vi "Digilens DLP Gen2 UI .vi"(11 "TopLevel In":refnum<class "TopLevel.lvclass">) -> (3 "TopLevel Out":refnum<class "TopLevel.lvclass">)   [LabVIEW 2022 SP3, in "TopLevel.lvclass"] (continued)
              frame "Stage Head3", "Stage Head3 2" {
                n548 = Unbundle By Name(w1508) -> ("Prime Names.Prime 3"=w1507:string)
              }
              frame "Stage Head4", "Stage Head4 2" {
                n549 = Unbundle By Name(w1513) -> ("Prime Names.Prime 4"=w1512:string)
              }
              frame "Stage Head5", "Stage Head5 2" {
                n550 = Unbundle By Name(w1518) -> ("Prime Names.Prime 5"=w1517:string)
              }
              frame "Stage Head6", "Stage Head6 2" {
                n551 = Unbundle By Name(w1523) -> ("Prime Names.Prime 6"=w1522:string)
              }
            }
            n552 = Unbundle By Name(w1488) -> ("Motor Controller"=w1475:refnum<class "Motor Controller.lvclass">, "Methods:Accessors:ConfigDict"=w1487:T16)
            n553 = call <vilib>:"Get Dynamic CVT Data.vi"("error in (no error)"=w1486, "default value (empty variant)"=w1483, "DataName"=w1485, "dCVT DVR"=w1487) -> ("error out"=w1482:errorcluster, "value"=w1484:variant)  [unwired: 4 in, 2 out]
            n554 = Variant To Data(error in=w1482, type=w1483, Variant=w1484) -> (data=w1481:T27, error out=w1474:errorcluster)
            n555 = Unbundle By Name(w1481) -> ("PrimingMode"=w1480:T13)
            n556 = Equal?(x=w1480, y=PurgeMode--Enum."Purge") -> (x = y?=w1466:bool)
            n557 = Select(t=w1468, s=w1466, f=w1467) -> (s? t:f=w1469:i32)
            n558 = Bundle By Name(cluster=T20 {"Motor Controller Parameter"=enum."Move Stage to Under PH1", "value"=11} ("SetExplicitMessage API Data"), "value"=w1469, "Motor Controller Parameter"=w1471) -> (w1470:T20)
            n559 = Bundle By Name(cluster=T23 {"Command"=enum."GetExplicitMessage", "Arguments"="", "Data"=variant} ("API Command Cluster"), "Command"=API_Command_Enum."SetExplicitMessage", "Data"=w1470) -> (w1478:T23)
            n560 = call-dynamic "GenerateAPIEvent_Motor Controller.vi"("error in (no error)"=w1474, "API Command Cluster"=w1478, "Motor Controller In"=w1475) -> ("error out"=w1473:errorcluster)  [unwired: 6 in, 2 out]
          }
          event "Prime Interval 1", "Prime Duration 1", "Prime Repeats 1", "Freq 1": Value Change {
            n561 = event-data() -> ()  [unwired: 1 in, 6 out]
            n562 = Unbundle By Name(w1534) -> ("TopLevel out"=w1524:refnum<class "TopLevel.lvclass">, "Methods:Accessors:ConfigDict"=w1532:T16, "Prime Names.Prime 1"=w1531:string)
            n563 = call <vilib>:"Get Dynamic CVT Data.vi"("error in (no error)"=w1530, "default value (empty variant)"=T27 {"Interval (s)"=0.1, "PurgeDuration (s)"=0.1, "Repeats"=0, "PrimingMode"=enum."Pre-Purge", "Head"=enum."1", "Frequency (Hz)"=0, "PrintWeight"=0.1} ("Pre Purge API Data"), "DataName"=w1531, "dCVT DVR"=w1532) -> ("error out"=w1529:errorcluster, "found"=w1526:bool, "value"=w1528:variant, "dCVT DVR out"=w1525:T16)  [unwired: 4 in]
            n564 = case shown="True" w1526 {
              tunnel: w1531 -> [_ w1550]
              tunnel: [w1538 w1546] -> w1535
              tunnel: w1534 -> [w1539 w1545]
              tunnel: [w1539 w1544] -> w1533
              tunnel: w1529 -> [w1538 w1555]
              tunnel: w1528 -> [_ w1554]
              tunnel: w1525 -> [_ w1552]
              tunnel: w1524 -> [_ w1543]
              frame False {
              }
              frame True {
                n565 = Variant To Data(error in=w1555, type=T27 {"Interval (s)"=0.1, "PurgeDuration (s)"=0.1, "Repeats"=0, "PrimingMode"=enum."Pre-Purge", "Head"=enum."1", "Frequency (Hz)"=0, "PrintWeight"=0.1} ("Pre Purge API Data"), Variant=w1554) -> (data=w1553:T27, error out=w1547:errorcluster)
                n566 = Bundle By Name(cluster=w1553, "Interval (s)"="Prime Interval 1", "PurgeDuration (s)"="Prime Duration 1", "Repeats"="Prime Repeats 1", "PrimingMode"="Prime Mode 1", "Frequency (Hz)"="Freq 1") -> (w1549:T27)
                n567 = call <vilib>:"Set Dynamic CVT Data.vi"("error in (no error)"=w1547, "value"=w1549, "DataName"=w1550, "dCVT DVR"=w1552) -> ("error out"=w1548:errorcluster, "dCVT DVR out"=w1551:T16)  [unwired: 5 in, 1 out]
                n568 = call-dynamic "Write ConfigDict.vi"("error in (no error)"=w1548, "ConfigDIct"=w1551, "TopLevel in"=w1543) -> ("error out"=w1546:errorcluster, "TopLevel out"=w1542:refnum<class "TopLevel.lvclass">)  [unwired: 7 in]
                n569 = Bundle By Name(cluster=w1545, "TopLevel out"=w1542) -> (w1544:T77)
              }
            }
          }
          event "Prime Interval 2", "Prime Duration 2", "Prime Repeats 2", "Freq 2": Value Change {
            n570 = event-data() -> ()  [unwired: 1 in, 6 out]
            n571 = Unbundle By Name(w1568) -> ("TopLevel out"=w1560:refnum<class "TopLevel.lvclass">, "Methods:Accessors:ConfigDict"=w1567:T16, "Prime Names.Prime 2"=w1566:string)
            n572 = call <vilib>:"Get Dynamic CVT Data.vi"("error in (no error)"=w1571, "default value (empty variant)"=T27 {"Interval (s)"=0.1, "PurgeDuration (s)"=0.1, "Repeats"=0, "PrimingMode"=enum."Pre-Purge", "Head"=enum."1", "Frequency (Hz)"=0, "PrintWeight"=0.1} ("Pre Purge API Data"), "DataName"=w1566, "dCVT DVR"=w1567) -> ("error out"=w1565:errorcluster, "found"=w1562:bool, "value"=w1564:variant, "dCVT DVR out"=w1561:T16)  [unwired: 4 in]
            n573 = case shown="True" w1562 {
              tunnel: w1566 -> [_ w1590]
              tunnel: [w1574 w1586] -> w1570
              tunnel: w1568 -> [w1575 w1585]
              tunnel: [w1575 w1584] -> w1569
              tunnel: w1565 -> [w1574 w1595]
              tunnel: w1564 -> [_ w1594]
              tunnel: w1561 -> [_ w1592]
              tunnel: w1560 -> [_ w1583]
              frame False {
              }
              frame True {
                n574 = Variant To Data(error in=w1595, type=T27 {"Interval (s)"=0.1, "PurgeDuration (s)"=0.1, "Repeats"=0, "PrimingMode"=enum."Pre-Purge", "Head"=enum."1", "Frequency (Hz)"=0, "PrintWeight"=0.1} ("Pre Purge API Data"), Variant=w1594) -> (data=w1593:T27, error out=w1587:errorcluster)
                n575 = Bundle By Name(cluster=w1593, "Interval (s)"="Prime Interval 2", "PurgeDuration (s)"="Prime Duration 2", "Repeats"="Prime Repeats 2", "PrimingMode"="Prime Mode 2", "Frequency (Hz)"="Freq 2") -> (w1589:T27)
                n576 = call <vilib>:"Set Dynamic CVT Data.vi"("error in (no error)"=w1587, "value"=w1589, "DataName"=w1590, "dCVT DVR"=w1592) -> ("error out"=w1588:errorcluster, "dCVT DVR out"=w1591:T16)  [unwired: 5 in, 1 out]
                n577 = call-dynamic "Write ConfigDict.vi"("error in (no error)"=w1588, "ConfigDIct"=w1591, "TopLevel in"=w1583) -> ("error out"=w1586:errorcluster, "TopLevel out"=w1582:refnum<class "TopLevel.lvclass">)  [unwired: 7 in]
                n578 = Bundle By Name(cluster=w1585, "TopLevel out"=w1582) -> (w1584:T77)
              }
            }
          }
          event "Prime Interval 3", "Prime Duration 3", "Prime Repeats 3", "Freq 3": Value Change {
            n579 = event-data() -> ()  [unwired: 1 in, 6 out]
            n580 = Unbundle By Name(w1604) -> ("TopLevel out"=w1596:refnum<class "TopLevel.lvclass">, "Methods:Accessors:ConfigDict"=w1603:T16, "Prime Names.Prime 3"=w1602:string)
            n581 = call <vilib>:"Get Dynamic CVT Data.vi"("error in (no error)"=w1607, "default value (empty variant)"=T27 {"Interval (s)"=0.1, "PurgeDuration (s)"=0.1, "Repeats"=0, "PrimingMode"=enum."Pre-Purge", "Head"=enum."1", "Frequency (Hz)"=0, "PrintWeight"=0.1} ("Pre Purge API Data"), "DataName"=w1602, "dCVT DVR"=w1603) -> ("error out"=w1601:errorcluster, "found"=w1598:bool, "value"=w1600:variant, "dCVT DVR out"=w1597:T16)  [unwired: 4 in]
            n582 = case shown="True" w1598 {
              tunnel: w1602 -> [_ w1626]
              tunnel: [w1610 w1622] -> w1606
              tunnel: w1604 -> [w1611 w1621]
              tunnel: [w1611 w1620] -> w1605
              tunnel: w1601 -> [w1610 w1631]
              tunnel: w1600 -> [_ w1630]
              tunnel: w1597 -> [_ w1628]
              tunnel: w1596 -> [_ w1619]
              frame False {
              }
              frame True {
                n583 = Variant To Data(error in=w1631, type=T27 {"Interval (s)"=0.1, "PurgeDuration (s)"=0.1, "Repeats"=0, "PrimingMode"=enum."Pre-Purge", "Head"=enum."1", "Frequency (Hz)"=0, "PrintWeight"=0.1} ("Pre Purge API Data"), Variant=w1630) -> (data=w1629:T27, error out=w1623:errorcluster)
                n584 = Bundle By Name(cluster=w1629, "Interval (s)"="Prime Interval 3", "PurgeDuration (s)"="Prime Duration 3", "Repeats"="Prime Repeats 3", "PrimingMode"="Prime Mode 3", "Frequency (Hz)"="Freq 3") -> (w1625:T27)
                n585 = call <vilib>:"Set Dynamic CVT Data.vi"("error in (no error)"=w1623, "value"=w1625, "DataName"=w1626, "dCVT DVR"=w1628) -> ("error out"=w1624:errorcluster, "dCVT DVR out"=w1627:T16)  [unwired: 5 in, 1 out]
                n586 = call-dynamic "Write ConfigDict.vi"("error in (no error)"=w1624, "ConfigDIct"=w1627, "TopLevel in"=w1619) -> ("error out"=w1622:errorcluster, "TopLevel out"=w1618:refnum<class "TopLevel.lvclass">)  [unwired: 7 in]
                n587 = Bundle By Name(cluster=w1621, "TopLevel out"=w1618) -> (w1620:T77)
              }
            }
          }
          event "Prime Interval 4", "Prime Duration 4", "Prime Repeats 4", "Freq 4": Value Change {
            n588 = event-data() -> ()  [unwired: 1 in, 6 out]
            n589 = Unbundle By Name(w1640) -> ("TopLevel out"=w1632:refnum<class "TopLevel.lvclass">, "Methods:Accessors:ConfigDict"=w1639:T16, "Prime Names.Prime 4"=w1638:string)
            n590 = call <vilib>:"Get Dynamic CVT Data.vi"("error in (no error)"=w1643, "default value (empty variant)"=T27 {"Interval (s)"=0.1, "PurgeDuration (s)"=0.1, "Repeats"=0, "PrimingMode"=enum."Pre-Purge", "Head"=enum."1", "Frequency (Hz)"=0, "PrintWeight"=0.1} ("Pre Purge API Data"), "DataName"=w1638, "dCVT DVR"=w1639) -> ("error out"=w1637:errorcluster, "found"=w1634:bool, "value"=w1636:variant, "dCVT DVR out"=w1633:T16)  [unwired: 4 in]
            n591 = case shown="True" w1634 {
              tunnel: w1638 -> [_ w1662]
              tunnel: [w1646 w1658] -> w1642
              tunnel: w1640 -> [w1647 w1657]
              tunnel: [w1647 w1656] -> w1641
              tunnel: w1637 -> [w1646 w1667]
              tunnel: w1636 -> [_ w1666]
              tunnel: w1633 -> [_ w1664]
              tunnel: w1632 -> [_ w1655]
              frame False {
              }
              frame True {
                n592 = Variant To Data(error in=w1667, type=T27 {"Interval (s)"=0.1, "PurgeDuration (s)"=0.1, "Repeats"=0, "PrimingMode"=enum."Pre-Purge", "Head"=enum."1", "Frequency (Hz)"=0, "PrintWeight"=0.1} ("Pre Purge API Data"), Variant=w1666) -> (data=w1665:T27, error out=w1659:errorcluster)
                n593 = Bundle By Name(cluster=w1665, "Interval (s)"="Prime Interval 4", "PurgeDuration (s)"="Prime Duration 4", "Repeats"="Prime Repeats 4", "PrimingMode"="Prime Mode 4", "Frequency (Hz)"="Freq 4") -> (w1661:T27)
                n594 = call <vilib>:"Set Dynamic CVT Data.vi"("error in (no error)"=w1659, "value"=w1661, "DataName"=w1662, "dCVT DVR"=w1664) -> ("error out"=w1660:errorcluster, "dCVT DVR out"=w1663:T16)  [unwired: 5 in, 1 out]
                n595 = call-dynamic "Write ConfigDict.vi"("error in (no error)"=w1660, "ConfigDIct"=w1663, "TopLevel in"=w1655) -> ("error out"=w1658:errorcluster, "TopLevel out"=w1654:refnum<class "TopLevel.lvclass">)  [unwired: 7 in]
                n596 = Bundle By Name(cluster=w1657, "TopLevel out"=w1654) -> (w1656:T77)
              }
            }
          }
          event "Prime Interavl 5", "Prime Duration 5", "Prime Repeats 5", "Freq 5": Value Change {
            n597 = event-data() -> ()  [unwired: 1 in, 6 out]
            n598 = Unbundle By Name(w1676) -> ("TopLevel out"=w1668:refnum<class "TopLevel.lvclass">, "Methods:Accessors:ConfigDict"=w1675:T16, "Prime Names.Prime 5"=w1674:string)
            n599 = call <vilib>:"Get Dynamic CVT Data.vi"("error in (no error)"=w1679, "default value (empty variant)"=T27 {"Interval (s)"=0.1, "PurgeDuration (s)"=0.1, "Repeats"=0, "PrimingMode"=enum."Pre-Purge", "Head"=enum."1", "Frequency (Hz)"=0, "PrintWeight"=0.1} ("Pre Purge API Data"), "DataName"=w1674, "dCVT DVR"=w1675) -> ("error out"=w1673:errorcluster, "found"=w1670:bool, "value"=w1672:variant, "dCVT DVR out"=w1669:T16)  [unwired: 4 in]
            n600 = case shown="True" w1670 {
              tunnel: w1674 -> [_ w1698]
              tunnel: [w1682 w1694] -> w1678
              tunnel: w1676 -> [w1683 w1693]
              tunnel: [w1683 w1692] -> w1677
              tunnel: w1673 -> [w1682 w1703]
              tunnel: w1672 -> [_ w1702]
              tunnel: w1669 -> [_ w1700]
              tunnel: w1668 -> [_ w1691]
              frame False {
              }
              frame True {
                n601 = Variant To Data(error in=w1703, type=T27 {"Interval (s)"=0.1, "PurgeDuration (s)"=0.1, "Repeats"=0, "PrimingMode"=enum."Pre-Purge", "Head"=enum."1", "Frequency (Hz)"=0, "PrintWeight"=0.1} ("Pre Purge API Data"), Variant=w1702) -> (data=w1701:T27, error out=w1695:errorcluster)
                n602 = Bundle By Name(cluster=w1701, "Interval (s)"="Prime Interavl 5", "PurgeDuration (s)"="Prime Duration 5", "Repeats"="Prime Repeats 5", "PrimingMode"="Prime Mode 5", "Frequency (Hz)"="Freq 5") -> (w1697:T27)
                n603 = call <vilib>:"Set Dynamic CVT Data.vi"("error in (no error)"=w1695, "value"=w1697, "DataName"=w1698, "dCVT DVR"=w1700) -> ("error out"=w1696:errorcluster, "dCVT DVR out"=w1699:T16)  [unwired: 5 in, 1 out]
                n604 = call-dynamic "Write ConfigDict.vi"("error in (no error)"=w1696, "ConfigDIct"=w1699, "TopLevel in"=w1691) -> ("error out"=w1694:errorcluster, "TopLevel out"=w1690:refnum<class "TopLevel.lvclass">)  [unwired: 7 in]
                n605 = Bundle By Name(cluster=w1693, "TopLevel out"=w1690) -> (w1692:T77)
              }
            }
          }
          event "Prime Interval 6", "Prime Duration 6", "Prime Repeats 6": Value Change {
            n606 = event-data() -> ()  [unwired: 1 in, 6 out]
            n607 = Unbundle By Name(w1712) -> ("TopLevel out"=w1704:refnum<class "TopLevel.lvclass">, "Methods:Accessors:ConfigDict"=w1711:T16, "Prime Names.Prime 6"=w1710:string)
            n608 = call <vilib>:"Get Dynamic CVT Data.vi"("error in (no error)"=w1715, "default value (empty variant)"=T27 {"Interval (s)"=0.1, "PurgeDuration (s)"=0.1, "Repeats"=0, "PrimingMode"=enum."Pre-Purge", "Head"=enum."1", "Frequency (Hz)"=0, "PrintWeight"=0.1} ("Pre Purge API Data"), "DataName"=w1710, "dCVT DVR"=w1711) -> ("error out"=w1709:errorcluster, "found"=w1706:bool, "value"=w1708:variant, "dCVT DVR out"=w1705:T16)  [unwired: 4 in]
            n609 = case shown="True" w1706 {
              tunnel: w1710 -> [_ w1734]
              tunnel: [w1719 w1730] -> w1714
              tunnel: w1709 -> [w1719 w1739]
              tunnel: w1708 -> [_ w1738]
              tunnel: w1705 -> [_ w1736]
              tunnel: w1704 -> [_ w1729]
              tunnel: w1712 -> [w1718 w1722]
              tunnel: [w1718 w1721] -> w1713
              frame False {
              }
              frame True {
                n610 = Variant To Data(error in=w1739, type=T27 {"Interval (s)"=0.1, "PurgeDuration (s)"=0.1, "Repeats"=0, "PrimingMode"=enum."Pre-Purge", "Head"=enum."1", "Frequency (Hz)"=0, "PrintWeight"=0.1} ("Pre Purge API Data"), Variant=w1738) -> (data=w1737:T27, error out=w1731:errorcluster)
                n611 = Bundle By Name(cluster=w1737, "Interval (s)"="Prime Interval 6", "PurgeDuration (s)"="Prime Duration 6", "Repeats"="Prime Repeats 6", "PrimingMode"="Prime Mode 6", "Frequency (Hz)"="Freq 6") -> (w1733:T27)
                n612 = call <vilib>:"Set Dynamic CVT Data.vi"("error in (no error)"=w1731, "value"=w1733, "DataName"=w1734, "dCVT DVR"=w1736) -> ("error out"=w1732:errorcluster, "dCVT DVR out"=w1735:T16)  [unwired: 5 in, 1 out]
                n613 = call-dynamic "Write ConfigDict.vi"("error in (no error)"=w1732, "ConfigDIct"=w1735, "TopLevel in"=w1729) -> ("error out"=w1730:errorcluster, "TopLevel out"=w1728:refnum<class "TopLevel.lvclass">)  [unwired: 7 in]
                n614 = Bundle By Name(cluster=w1722, "TopLevel out"=w1728) -> (w1721:T77)
              }
            }
          }
          event "Print": Value Change {
            n615 = event-data() -> ()  [unwired: 1 in, 6 out]
            n616 = Bundle By Name(cluster=T28 {"Command File Path"=path "", "No. of Print Repeats"=1, "HomeOnComplete"=FALSE}, "Command File Path"="Command File Path", "No. of Print Repeats"="Print Passes", "HomeOnComplete"="HomeOnComplete") -> (w1744:T28)
            n617 = Bundle By Name(cluster=T29 {"Command"=enum."Execute Printer Commands", "Arguments"="", "Data"=variant} ("API Command Cluster"), "Command"=API_Command_Enum."Execute Printer Commands", "Data"=w1744) -> (w1748:T29)
            n618 = call-dynamic "GenerateAPIEvent_TopLevel.vi"("Wait (F)"=FALSE, "error in (no error)"=w1750, "API Command Cluster"=w1748, "TopLevel in"=w1752) -> ("error out"=w1751:errorcluster, "TopLevel out"=w1753:refnum<class "TopLevel.lvclass">)  [unwired: 6 in]
          }
          event "IdlePrint": Value Change {
            n619 = event-data() -> ("NewVal"=w1758:bool)  [unwired: 1 in, 5 out]
            n620 = case shown="True" w1758 {
              tunnel: [API_Command_Enum."StopIdlePrintCycle" ("Command") API_Command_Enum."ExecuteIdlePrintCycle" ("Command")] -> w1762
              tunnel: [w1771 w1779] -> w1761
              tunnel: w1758 -> [_ w1776]
              tunnel: ["UI: SetUIControlsState>>enable" ("State(s) in Front (\"\")") "UI: SetUIControlsState>>disable" ("State(s) in Front (\"\")")] -> w1755
              frame False {
                n621 = Bundle By Name(cluster=T30 {"Command File Path"=path "", "IdleMode"=FALSE, "IdleCycleInterval(s)"=0.0} ("Cluster"), "IdleMode"=FALSE) -> (w1771:T30)
              }
              frame True {
                n622 = property on="Command File Path" class="Path"() -> ("Value"=w1775:path)  [unwired: 2 in, 2 out]
                n623 = Bundle By Name(cluster=T30 {"Command File Path"=path "", "IdleMode"=FALSE, "IdleCycleInterval(s)"=0.0} ("Cluster"), "Command File Path"=w1775, "IdleMode"=w1776, "IdleCycleInterval(s)"="Idle Intervals (s)") -> (w1779:T30)
              }
            }
            n624 = Bundle By Name(cluster=T29 {"Command"=enum."Execute Printer Commands", "Arguments"="", "Data"=variant} ("API Command Cluster"), "Command"=w1762, "Data"=w1761) -> (w1763:T29)
            n625 = call-dynamic "GenerateAPIEvent_TopLevel.vi"("Wait (F)"=FALSE, "error in (no error)"=w1765, "API Command Cluster"=w1763, "TopLevel in"=w1767) -> ("error out"=w1766:errorcluster, "TopLevel out"=w1768:refnum<class "TopLevel.lvclass">)  [unwired: 6 in]
            n626 = call <vilib>:"Add State(s) to Queue__JKI_lib_State_Machine.vi"("State(s) in Front (\"\")"=w1755, "State(s) in (\"\")"=w1756) -> ("States Out"=w1757:string)  [unwired: 13 in]
          }
          event User Event {
            n627 = event-data() -> ()  [unwired: 1 in, 6 out]
            n628 = Unbundle By Name(w1788) -> ("GIS Printer"=w1787:refnum<class "GIS Printer.lvclass">)
            n629 = call-dynamic "GetTCPCommandsResponses_GIS Printer.vi"("error in (no error)"=w1785, "gis in"=w1787) -> ("error out"=w1786:errorcluster, "TCP Commands & Responses"=w1784:string[][])  [unwired: 7 in, 1 out]
            n630 = property on="TCP Commands & Responses" class="MCListbox (strict)"("ItemNames"=w1784) -> ()  [unwired: 2 in, 2 out]
            n631 = call <vilib>:"Add State(s) to Queue__JKI_lib_State_Machine.vi"("State(s) in Front (\"\")"="UI: Update Stage Busy", "State(s) in (\"\")"=w1782) -> ("States Out"=w1783:string)  [unwired: 13 in]
          }
          event "Meniscus Valve Open - R1": Value Change {
            n632 = event-data() -> ()  [unwired: 1 in, 6 out]
            n633 = Unbundle By Name(w1796) -> ("DAQ"=w1791:refnum<class "DAQ.lvclass">, "IO"=w1795:refnum<class "IO.lvclass">)
            n634 = disable-structure shown="Enabled" {
              disable-tunnel: w1795 -> [w1803 _]
              disable-tunnel: "Meniscus Valve Open - R1" -> [w1802 w1808]
              disable-tunnel: [w1801 w1811] -> w1793
              disable-tunnel: w1792 -> [w1800 w1810]
              disable-tunnel: w1791 -> [_ w1809]
              disable-tunnel: ICP2-DO_Channel_Names."Meniscus Valve Open - R1" ("DO Channel") -> [w1799 w1807]
              disable-tunnel: [_ w1805] -> _
              frame Disabled {
                n635 = call-dynamic "Set ICP2-DO Changed bit.vi"("error in (no error)"=w1800, "Value"=w1802, "DO Channel"=w1799, "IO in"=w1803) -> ("error out"=w1801:errorcluster)  [unwired: 6 in, 1 out]
              }
              frame Enabled {
                n636 = Format Into String(format string="%s", w1807) -> (resulting string=w1806:string)  [unwired: 2 in, 1 out]
                n637 = call "Set DO State (manual mode).vi"("error in (no error)"=w1810, "State"=w1808, "DO IOName"=w1806, "DAQ"=w1809) -> ("error out"=w1811:errorcluster, "DAQ"=w1805:refnum<class "DAQ.lvclass">)  [unwired: 6 in]
              }
            }
          }
          event "Meniscus Valve Open - R2": Value Change {
            n638 = event-data() -> ()  [unwired: 1 in, 6 out]
            n639 = Unbundle By Name(w1817) -> ("DAQ"=w1812:refnum<class "DAQ.lvclass">, "IO"=w1816:refnum<class "IO.lvclass">)
            n640 = disable-structure shown="Enabled" {
              disable-tunnel: ICP2-DO_Channel_Names."Meniscus Valve Open - R2" ("DO Channel") -> [w1825 w1826]
              disable-tunnel: w1816 -> [w1824 _]
              disable-tunnel: [w1823 w1830] -> w1815
              disable-tunnel: w1814 -> [w1822 w1831]
              disable-tunnel: "Meniscus Valve Open - R2" -> [w1821 w1829]
              disable-tunnel: w1812 -> [_ w1828]
              frame Disabled {
                n641 = call-dynamic "Set ICP2-DO Changed bit.vi"("error in (no error)"=w1822, "Value"=w1821, "DO Channel"=w1825, "IO in"=w1824) -> ("error out"=w1823:errorcluster)  [unwired: 6 in, 1 out]
              }
              frame Enabled {
                n642 = Format Into String(format string="%s", w1826) -> (resulting string=w1832:string)  [unwired: 2 in, 1 out]
                n643 = call "Set DO State (manual mode).vi"("error in (no error)"=w1831, "State"=w1829, "DO IOName"=w1832, "DAQ"=w1828) -> ("error out"=w1830:errorcluster)  [unwired: 6 in, 1 out]
              }
            }
          }
          event "Meniscus Valve Open - R3": Value Change {
            n644 = event-data() -> ()  [unwired: 1 in, 6 out]
            n645 = Unbundle By Name(w1838) -> ("DAQ"=w1833:refnum<class "DAQ.lvclass">, "IO"=w1837:refnum<class "IO.lvclass">)
            n646 = disable-structure shown="Enabled" {
              disable-tunnel: ICP2-DO_Channel_Names."Meniscus Valve Open - R3" ("DO Channel") -> [w1846 w1847]
              disable-tunnel: w1837 -> [w1845 _]
              disable-tunnel: [w1844 w1850] -> w1836
              disable-tunnel: w1835 -> [w1843 w1851]
              disable-tunnel: "Meniscus Valve Open - R3" -> [w1842 w1849]
              disable-tunnel: w1833 -> [_ w1848]
              frame Disabled {
                n647 = call-dynamic "Set ICP2-DO Changed bit.vi"("error in (no error)"=w1843, "Value"=w1842, "DO Channel"=w1846, "IO in"=w1845) -> ("error out"=w1844:errorcluster)  [unwired: 6 in, 1 out]
              }
              frame Enabled {
                n648 = Format Into String(format string="%s", w1847) -> (resulting string=w1853:string)  [unwired: 2 in, 1 out]
                n649 = call "Set DO State (manual mode).vi"("error in (no error)"=w1851, "State"=w1849, "DO IOName"=w1853, "DAQ"=w1848) -> ("error out"=w1850:errorcluster)  [unwired: 6 in, 1 out]
              }
            }
          }
          event "Meniscus Valve Open - R4": Value Change {
            n650 = event-data() -> ()  [unwired: 1 in, 6 out]
            n651 = Unbundle By Name(w1859) -> ("DAQ"=w1854:refnum<class "DAQ.lvclass">, "IO"=w1858:refnum<class "IO.lvclass">)
            n652 = disable-structure shown="Enabled" {
              disable-tunnel: ICP2-DO_Channel_Names."Meniscus Valve Open - R4" ("DO Channel") -> [w1867 w1868]
              disable-tunnel: w1858 -> [w1866 _]
              disable-tunnel: [w1865 w1871] -> w1857
              disable-tunnel: w1856 -> [w1864 w1872]
              disable-tunnel: "Meniscus Valve Open - R4" -> [w1863 w1870]
              disable-tunnel: w1854 -> [_ w1869]
              frame Disabled {
                n653 = call-dynamic "Set ICP2-DO Changed bit.vi"("error in (no error)"=w1864, "Value"=w1863, "DO Channel"=w1867, "IO in"=w1866) -> ("error out"=w1865:errorcluster)  [unwired: 6 in, 1 out]
              }
              frame Enabled {
                n654 = Format Into String(format string="%s", w1868) -> (resulting string=w1874:string)  [unwired: 2 in, 1 out]
                n655 = call "Set DO State (manual mode).vi"("error in (no error)"=w1872, "State"=w1870, "DO IOName"=w1874, "DAQ"=w1869) -> ("error out"=w1871:errorcluster)  [unwired: 6 in, 1 out]
              }
            }
          }
          event "Meniscus Valve Open - R5": Value Change {
            n656 = event-data() -> ()  [unwired: 1 in, 6 out]
            n657 = Unbundle By Name(w1880) -> ("DAQ"=w1875:refnum<class "DAQ.lvclass">, "IO"=w1879:refnum<class "IO.lvclass">)
            n658 = disable-structure shown="Enabled" {
              disable-tunnel: ICP2-DO_Channel_Names."Meniscus Valve Open - R5" ("DO Channel") -> [w1888 w1893]
              disable-tunnel: w1879 -> [w1887 _]
              disable-tunnel: [w1886 w1890] -> w1878
              disable-tunnel: w1877 -> [w1885 w1892]
              disable-tunnel: "Meniscus Valve Open - R5" -> [w1884 w1889]
              disable-tunnel: w1875 -> [_ w1894]
              frame Disabled {
                n659 = call-dynamic "Set ICP2-DO Changed bit.vi"("error in (no error)"=w1885, "Value"=w1884, "DO Channel"=w1888, "IO in"=w1887) -> ("error out"=w1886:errorcluster)  [unwired: 6 in, 1 out]
              }
              frame Enabled {
                n660 = Format Into String(format string="%s", error in=w1892, w1893) -> (resulting string=w1896:string, error out=w1891:errorcluster)  [unwired: 1 in]
                n661 = call "Set DO State (manual mode).vi"("error in (no error)"=w1891, "State"=w1889, "DO IOName"=w1896, "DAQ"=w1894) -> ("error out"=w1890:errorcluster)  [unwired: 6 in, 1 out]
              }
            }
          }
          event "Meniscus Valve Open - R6": Value Change {
            n662 = event-data() -> ()  [unwired: 1 in, 6 out]
            n663 = Unbundle By Name(w1902) -> ("DAQ"=w1897:refnum<class "DAQ.lvclass">, "IO"=w1901:refnum<class "IO.lvclass">)
            n664 = disable-structure shown="Enabled" {
              disable-tunnel: ICP2-DO_Channel_Names."Meniscus Valve Open - R6" ("DO Channel") -> [w1910 w1913]
              disable-tunnel: w1901 -> [w1909 _]
              disable-tunnel: [w1908 w1911] -> w1900
              disable-tunnel: w1899 -> [w1907 w1912]
              disable-tunnel: "Meniscus Valve Open - R6" -> [w1906 w1915]
              disable-tunnel: w1897 -> [_ w1914]
              frame Disabled {
                n665 = call-dynamic "Set ICP2-DO Changed bit.vi"("error in (no error)"=w1907, "Value"=w1906, "DO Channel"=w1910, "IO in"=w1909) -> ("error out"=w1908:errorcluster)  [unwired: 6 in, 1 out]
              }
              frame Enabled {
                n666 = Format Into String(format string="%s", w1913) -> (resulting string=w1917:string)  [unwired: 2 in, 1 out]
                n667 = call "Set DO State (manual mode).vi"("error in (no error)"=w1912, "State"=w1915, "DO IOName"=w1917, "DAQ"=w1914) -> ("error out"=w1911:errorcluster)  [unwired: 6 in, 1 out]
              }
            }
          }
          event "Ink Flow Valve Open - R1": Value Change {
            n668 = event-data() -> ()  [unwired: 1 in, 6 out]
            n669 = Unbundle By Name(w1923) -> ("DAQ"=w1918:refnum<class "DAQ.lvclass">, "IO"=w1922:refnum<class "IO.lvclass">)
            n670 = disable-structure shown="Enabled" {
              disable-tunnel: ICP2-DO_Channel_Names."Ink Flow Valve Open - R1" ("DO Channel") -> [w1931 w1945]
              disable-tunnel: w1922 -> [w1930 _]
              disable-tunnel: [w1929 w1933] -> w1921
              disable-tunnel: w1920 -> [w1928 w1946]
              disable-tunnel: "Ink Flow Valve Open - R1" -> [w1927 w1932]
              disable-tunnel: w1918 -> [_ w1944]
              frame Disabled {
                n671 = call-dynamic "Set ICP2-DO Changed bit.vi"("error in (no error)"=w1928, "Value"=w1927, "DO Channel"=w1931, "IO in"=w1930) -> ("error out"=w1929:errorcluster)  [unwired: 6 in, 1 out]
              }
              frame Enabled {
                n672 = Format Into String(format string="%s", w1945) -> (resulting string=w1948:string)  [unwired: 2 in, 1 out]
                n673 = call "Set DO State (manual mode).vi"("error in (no error)"=w1946, "State"=w1932, "DO IOName"=w1948, "DAQ"=w1944) -> ("error out"=w1939:errorcluster, "DAQ"=w1940:refnum<class "DAQ.lvclass">)  [unwired: 6 in]
                n674 = Format Into String(format string="%s", ICP2-DO_Channel_Names."SW_LED - Ink Valve - R1" ("DO Channel")) -> (resulting string=w1943:string)  [unwired: 2 in, 1 out]
                n675 = call "Set DO State (automation mode).vi"("error in (no error)"=w1939, "State"=w1932, "DO IOName"=w1943, "DAQ"=w1940) -> ("error out"=w1934:errorcluster, "DAQ"=w1935:refnum<class "DAQ.lvclass">)  [unwired: 6 in]
                n676 = Format Into String(format string="%s", ICP2-DO_Channel_Names."Recirc Pump On - R1" ("DO Channel")) -> (resulting string=w1936:string)  [unwired: 2 in, 1 out]
                n677 = call "Set DO State (automation mode).vi"("error in (no error)"=w1934, "State"=w1932, "DO IOName"=w1936, "DAQ"=w1935) -> ("error out"=w1933:errorcluster)  [unwired: 6 in, 1 out]
              }
            }
          }
          event "Ink Flow Valve Open - R2": Value Change {
            n678 = event-data() -> ()  [unwired: 1 in, 6 out]
            n679 = Unbundle By Name(w1954) -> ("DAQ"=w1949:refnum<class "DAQ.lvclass">, "IO"=w1953:refnum<class "IO.lvclass">)
            n680 = disable-structure shown="Enabled" {
              disable-tunnel: ICP2-DO_Channel_Names."Ink Flow Valve Open - R2" ("DO Channel") -> [w1962 w1976]
              disable-tunnel: w1953 -> [w1961 _]
              disable-tunnel: [w1960 w1966] -> w1952
              disable-tunnel: w1951 -> [w1959 w1978]
              disable-tunnel: "Ink Flow Valve Open - R2" -> [w1958 w1965]
              disable-tunnel: w1949 -> [_ w1977]
              frame Disabled {
                n681 = call-dynamic "Set ICP2-DO Changed bit.vi"("error in (no error)"=w1959, "Value"=w1958, "DO Channel"=w1962, "IO in"=w1961) -> ("error out"=w1960:errorcluster)  [unwired: 6 in, 1 out]
              }
              frame Enabled {
                n682 = Format Into String(format string="%s", w1976) -> (resulting string=w1980:string)  [unwired: 2 in, 1 out]
                n683 = call "Set DO State (manual mode).vi"("error in (no error)"=w1978, "State"=w1965, "DO IOName"=w1980, "DAQ"=w1977) -> ("error out"=w1971:errorcluster, "DAQ"=w1972:refnum<class "DAQ.lvclass">)  [unwired: 6 in]
                n684 = Format Into String(format string="%s", ICP2-DO_Channel_Names."SW_LED - Ink Valve - R2" ("DO Channel")) -> (resulting string=w1975:string)  [unwired: 2 in, 1 out]
                n685 = call "Set DO State (automation mode).vi"("error in (no error)"=w1971, "State"=w1965, "DO IOName"=w1975, "DAQ"=w1972) -> ("error out"=w1964:errorcluster, "DAQ"=w1967:refnum<class "DAQ.lvclass">)  [unwired: 6 in]
                n686 = Format Into String(format string="%s", error in=w1964, ICP2-DO_Channel_Names."Recirc Pump On - R2" ("DO Channel")) -> (resulting string=w1968:string, error out=w1963:errorcluster)  [unwired: 1 in]
                n687 = call "Set DO State (automation mode).vi"("error in (no error)"=w1963, "State"=w1965, "DO IOName"=w1968, "DAQ"=w1967) -> ("error out"=w1966:errorcluster)  [unwired: 6 in, 1 out]
              }
            }
          }
          event "Ink Flow Valve Open - R3": Value Change {
            n688 = event-data() -> ()  [unwired: 1 in, 6 out]
            n689 = Unbundle By Name(w1986) -> ("DAQ"=w1981:refnum<class "DAQ.lvclass">, "IO"=w1985:refnum<class "IO.lvclass">)
            n690 = disable-structure shown="Enabled" {
              disable-tunnel: ICP2-DO_Channel_Names."Ink Flow Valve Open - R3" ("DO Channel") -> [w1994 w2010]
              disable-tunnel: w1985 -> [w1993 _]
              disable-tunnel: [w1992 w1998] -> w1984
              disable-tunnel: w1983 -> [w1991 w2011]
              disable-tunnel: "Ink Flow Valve Open - R3" -> [w1990 w1995]
              disable-tunnel: w1981 -> [_ w2009]
              frame Disabled {
                n691 = call-dynamic "Set ICP2-DO Changed bit.vi"("error in (no error)"=w1991, "Value"=w1990, "DO Channel"=w1994, "IO in"=w1993) -> ("error out"=w1992:errorcluster)  [unwired: 6 in, 1 out]
              }
              frame Enabled {
                n692 = Format Into String(format string="%s", w2010) -> (resulting string=w2013:string)  [unwired: 2 in, 1 out]
                n693 = call "Set DO State (manual mode).vi"("error in (no error)"=w2011, "State"=w1995, "DO IOName"=w2013, "DAQ"=w2009) -> ("error out"=w2005:errorcluster, "DAQ"=w2003:refnum<class "DAQ.lvclass">)  [unwired: 6 in]
                n694 = Format Into String(format string="%s", error in=w2005, ICP2-DO_Channel_Names."SW_LED - Ink Valve - R3" ("DO Channel")) -> (resulting string=w2008:string, error out=w2004:errorcluster)  [unwired: 1 in]
                n695 = call "Set DO State (automation mode).vi"("error in (no error)"=w2004, "State"=w1995, "DO IOName"=w2008, "DAQ"=w2003) -> ("error out"=w1997:errorcluster, "DAQ"=w1999:refnum<class "DAQ.lvclass">)  [unwired: 6 in]
                n696 = Format Into String(format string="%s", error in=w1997, ICP2-DO_Channel_Names."Recirc Pump On - R3" ("DO Channel")) -> (resulting string=w2000:string, error out=w1996:errorcluster)  [unwired: 1 in]
                n697 = call "Set DO State (automation mode).vi"("error in (no error)"=w1996, "State"=w1995, "DO IOName"=w2000, "DAQ"=w1999) -> ("error out"=w1998:errorcluster)  [unwired: 6 in, 1 out]
              }
            }
          }
          event "Ink Flow Valve Open - R4": Value Change {
            n698 = event-data() -> ()  [unwired: 1 in, 6 out]
            n699 = Unbundle By Name(w2019) -> ("DAQ"=w2014:refnum<class "DAQ.lvclass">, "IO"=w2018:refnum<class "IO.lvclass">)
            n700 = disable-structure shown="Enabled" {
              disable-tunnel: ICP2-DO_Channel_Names."Ink Flow Valve Open - R4" ("DO Channel") -> [w2027 w2042]
              disable-tunnel: w2018 -> [w2026 _]
              disable-tunnel: [w2025 w2029] -> w2017
              disable-tunnel: w2016 -> [w2024 w2044]
              disable-tunnel: "Ink Flow Valve Open - R4" -> [w2023 w2028]
              disable-tunnel: w2014 -> [_ w2043]
              frame Disabled {
                n701 = call-dynamic "Set ICP2-DO Changed bit.vi"("error in (no error)"=w2024, "Value"=w2023, "DO Channel"=w2027, "IO in"=w2026) -> ("error out"=w2025:errorcluster)  [unwired: 6 in, 1 out]
              }
              frame Enabled {
                n702 = Format Into String(format string="%s", w2042) -> (resulting string=w2046:string)  [unwired: 2 in, 1 out]
                n703 = call "Set DO State (manual mode).vi"("error in (no error)"=w2044, "State"=w2028, "DO IOName"=w2046, "DAQ"=w2043) -> ("error out"=w2036:errorcluster, "DAQ"=w2038:refnum<class "DAQ.lvclass">)  [unwired: 6 in]
                n704 = Format Into String(format string="%s", error in=w2036, ICP2-DO_Channel_Names."SW_LED - Ink Valve - R4" ("DO Channel")) -> (resulting string=w2041:string, error out=w2037:errorcluster)  [unwired: 1 in]
                n705 = call "Set DO State (automation mode).vi"("error in (no error)"=w2037, "State"=w2028, "DO IOName"=w2041, "DAQ"=w2038) -> ("error out"=w2030:errorcluster, "DAQ"=w2032:refnum<class "DAQ.lvclass">)  [unwired: 6 in]
                n706 = Format Into String(format string="%s", error in=w2030, ICP2-DO_Channel_Names."Recirc Pump On - R4" ("DO Channel")) -> (resulting string=w2033:string, error out=w2031:errorcluster)  [unwired: 1 in]
                n707 = call "Set DO State (automation mode).vi"("error in (no error)"=w2031, "State"=w2028, "DO IOName"=w2033, "DAQ"=w2032) -> ("error out"=w2029:errorcluster)  [unwired: 6 in, 1 out]
              }
            }
          }
          event "Ink Flow Valve Open - R5": Value Change {
            n708 = event-data() -> ()  [unwired: 1 in, 6 out]
            n709 = Unbundle By Name(w2052) -> ("DAQ"=w2047:refnum<class "DAQ.lvclass">, "IO"=w2051:refnum<class "IO.lvclass">)
            n710 = disable-structure shown="Enabled" {
              disable-tunnel: ICP2-DO_Channel_Names."Ink Flow Valve Open - R5" ("DO Channel") -> [w2060 w2077]
              disable-tunnel: w2051 -> [w2059 _]
              disable-tunnel: [w2058 w2064] -> w2050
              disable-tunnel: w2049 -> [w2057 w2075]
              disable-tunnel: "Ink Flow Valve Open - R5" -> [w2056 w2063]
              disable-tunnel: w2047 -> [_ w2076]
              frame Disabled {
                n711 = call-dynamic "Set ICP2-DO Changed bit.vi"("error in (no error)"=w2057, "Value"=w2056, "DO Channel"=w2060, "IO in"=w2059) -> ("error out"=w2058:errorcluster)  [unwired: 6 in, 1 out]
              }
              frame Enabled {
                n712 = Format Into String(format string="%s", w2077) -> (resulting string=w2079:string)  [unwired: 2 in, 1 out]
                n713 = call "Set DO State (manual mode).vi"("error in (no error)"=w2075, "State"=w2063, "DO IOName"=w2079, "DAQ"=w2076) -> ("error out"=w2069:errorcluster, "DAQ"=w2071:refnum<class "DAQ.lvclass">)  [unwired: 6 in]
                n714 = Format Into String(format string="%s", error in=w2069, ICP2-DO_Channel_Names."SW_LED - Ink Valve - R5" ("DO Channel")) -> (resulting string=w2074:string, error out=w2070:errorcluster)  [unwired: 1 in]
                n715 = call "Set DO State (automation mode).vi"("error in (no error)"=w2070, "State"=w2063, "DO IOName"=w2074, "DAQ"=w2071) -> ("error out"=w2062:errorcluster, "DAQ"=w2065:refnum<class "DAQ.lvclass">)  [unwired: 6 in]
                n716 = Format Into String(format string="%s", error in=w2062, ICP2-DO_Channel_Names."Recirc Pump On - R5" ("DO Channel")) -> (resulting string=w2066:string, error out=w2061:errorcluster)  [unwired: 1 in]
                n717 = call "Set DO State (automation mode).vi"("error in (no error)"=w2061, "State"=w2063, "DO IOName"=w2066, "DAQ"=w2065) -> ("error out"=w2064:errorcluster)  [unwired: 6 in, 1 out]
              }
            }
          }
          event "Ink Flow Valve Open - R6": Value Change {
            n718 = event-data() -> ()  [unwired: 1 in, 6 out]
            n719 = Unbundle By Name(w2085) -> ("DAQ"=w2080:refnum<class "DAQ.lvclass">, "IO"=w2084:refnum<class "IO.lvclass">)
            n720 = disable-structure shown="Enabled" {
              disable-tunnel: ICP2-DO_Channel_Names."Ink Flow Valve Open - R6" ("DO Channel") -> [w2093 w2109]
              disable-tunnel: w2084 -> [w2092 _]
              disable-tunnel: [w2091 w2097] -> w2083
              disable-tunnel: w2082 -> [w2090 w2110]
              disable-tunnel: "Ink Flow Valve Open - R6" -> [w2089 w2096]
              disable-tunnel: w2080 -> [_ w2108]
              frame Disabled {
                n721 = call-dynamic "Set ICP2-DO Changed bit.vi"("error in (no error)"=w2090, "Value"=w2089, "DO Channel"=w2093, "IO in"=w2092) -> ("error out"=w2091:errorcluster)  [unwired: 6 in, 1 out]
              }
              frame Enabled {
                n722 = Format Into String(format string="%s", w2109) -> (resulting string=w2112:string)  [unwired: 2 in, 1 out]
                n723 = call "Set DO State (manual mode).vi"("error in (no error)"=w2110, "State"=w2096, "DO IOName"=w2112, "DAQ"=w2108) -> ("error out"=w2102:errorcluster, "DAQ"=w2105:refnum<class "DAQ.lvclass">)  [unwired: 6 in]
                n724 = Format Into String(format string="%s", error in=w2102, ICP2-DO_Channel_Names."SW_LED - Ink Valve - R6" ("DO Channel")) -> (resulting string=w2104:string, error out=w2103:errorcluster)  [unwired: 1 in]
                n725 = call "Set DO State (automation mode).vi"("error in (no error)"=w2103, "State"=w2096, "DO IOName"=w2104, "DAQ"=w2105) -> ("error out"=w2095:errorcluster, "DAQ"=w2098:refnum<class "DAQ.lvclass">)  [unwired: 6 in]
                n726 = Format Into String(format string="%s", error in=w2095, ICP2-DO_Channel_Names."Recirc Pump On - R6" ("DO Channel")) -> (resulting string=w2099:string, error out=w2094:errorcluster)  [unwired: 1 in]
                n727 = call "Set DO State (automation mode).vi"("error in (no error)"=w2094, "State"=w2096, "DO IOName"=w2099, "DAQ"=w2098) -> ("error out"=w2097:errorcluster)  [unwired: 6 in, 1 out]
              }
            }
          }
          event "SW_LED - Ink Valve - R1": Value Change {
            n728 = event-data() -> ()  [unwired: 1 in, 6 out]
            n729 = Unbundle By Name(w2118) -> ("DAQ"=w2113:refnum<class "DAQ.lvclass">, "IO"=w2117:refnum<class "IO.lvclass">)
            n730 = disable-structure shown="Enabled" {
              disable-tunnel: ICP2-DO_Channel_Names."SW_LED - Ink Valve - R1" ("DO Channel") -> [w2126 w2141]
              disable-tunnel: w2117 -> [w2125 _]
              disable-tunnel: [w2124 w2127] -> w2116
              disable-tunnel: w2115 -> [w2123 w2142]
              disable-tunnel: "SW_LED - Ink Valve - R1" -> [w2122 w2129]
              disable-tunnel: w2113 -> [_ w2140]
              frame Disabled {
                n731 = call-dynamic "Set ICP2-DO Changed bit.vi"("error in (no error)"=w2123, "Value"=w2122, "DO Channel"=w2126, "IO in"=w2125) -> ("error out"=w2124:errorcluster)  [unwired: 6 in, 1 out]
              }
              frame Enabled {
                n732 = Format Into String(format string="%s", w2141) -> (resulting string=w2144:string)  [unwired: 2 in, 1 out]
                n733 = call "Set DO State (manual mode).vi"("error in (no error)"=w2142, "State"=w2129, "DO IOName"=w2144, "DAQ"=w2140) -> ("error out"=w2135:errorcluster, "DAQ"=w2134:refnum<class "DAQ.lvclass">)  [unwired: 6 in]
                n734 = Format Into String(format string="%s", error in=w2135, ICP2-DO_Channel_Names."Ink Flow Valve Open - R1" ("DO Channel")) -> (resulting string=w2139:string, error out=w2136:errorcluster)  [unwired: 1 in]
                n735 = call "Set DO State (automation mode).vi"("error in (no error)"=w2136, "State"=w2129, "DO IOName"=w2139, "DAQ"=w2134) -> ("error out"=w2128:errorcluster, "DAQ"=w2130:refnum<class "DAQ.lvclass">)  [unwired: 6 in]
                n736 = Format Into String(format string="%s", ICP2-DO_Channel_Names."Recirc Pump On - R1" ("DO Channel")) -> (resulting string=w2131:string)  [unwired: 2 in, 1 out]
                n737 = call "Set DO State (automation mode).vi"("error in (no error)"=w2128, "State"=w2129, "DO IOName"=w2131, "DAQ"=w2130) -> ("error out"=w2127:errorcluster)  [unwired: 6 in, 1 out]
              }
            }
          }
          event "SW_LED - Ink Valve - R2": Value Change {
            n738 = event-data() -> ()  [unwired: 1 in, 6 out]
            n739 = Unbundle By Name(w2150) -> ("DAQ"=w2145:refnum<class "DAQ.lvclass">, "IO"=w2149:refnum<class "IO.lvclass">)
            n740 = disable-structure shown="Enabled" {
              disable-tunnel: ICP2-DO_Channel_Names."SW_LED - Ink Valve - R2" ("DO Channel") -> [w2158 w2172]
              disable-tunnel: w2149 -> [w2157 _]
              disable-tunnel: [w2156 w2159] -> w2148
              disable-tunnel: w2147 -> [w2155 w2174]
              disable-tunnel: "SW_LED - Ink Valve - R2" -> [w2154 w2161]
              disable-tunnel: w2145 -> [_ w2173]
              frame Disabled {
                n741 = call-dynamic "Set ICP2-DO Changed bit.vi"("error in (no error)"=w2155, "Value"=w2154, "DO Channel"=w2158, "IO in"=w2157) -> ("error out"=w2156:errorcluster)  [unwired: 6 in, 1 out]
              }
              frame Enabled {
                n742 = Format Into String(format string="%s", w2172) -> (resulting string=w2176:string)  [unwired: 2 in, 1 out]
                n743 = call "Set DO State (manual mode).vi"("error in (no error)"=w2174, "State"=w2161, "DO IOName"=w2176, "DAQ"=w2173) -> ("error out"=w2166:errorcluster, "DAQ"=w2167:refnum<class "DAQ.lvclass">)  [unwired: 6 in]
                n744 = Format Into String(format string="%s", error in=w2166, ICP2-DO_Channel_Names."Ink Flow Valve Open - R2" ("DO Channel")) -> (resulting string=w2171:string, error out=w2168:errorcluster)  [unwired: 1 in]
                n745 = call "Set DO State (automation mode).vi"("error in (no error)"=w2168, "State"=w2161, "DO IOName"=w2171, "DAQ"=w2167) -> ("error out"=w2160:errorcluster, "DAQ"=w2162:refnum<class "DAQ.lvclass">)  [unwired: 6 in]
                n746 = Format Into String(format string="%s", ICP2-DO_Channel_Names."Recirc Pump On - R2" ("DO Channel")) -> (resulting string=w2163:string)  [unwired: 2 in, 1 out]
                n747 = call "Set DO State (automation mode).vi"("error in (no error)"=w2160, "State"=w2161, "DO IOName"=w2163, "DAQ"=w2162) -> ("error out"=w2159:errorcluster)  [unwired: 6 in, 1 out]
              }
            }
          }
          event "SW_LED - Ink Valve - R3": Value Change {
            n748 = event-data() -> ()  [unwired: 1 in, 6 out]
            n749 = Unbundle By Name(w2182) -> ("DAQ"=w2177:refnum<class "DAQ.lvclass">, "IO"=w2181:refnum<class "IO.lvclass">)
            n750 = disable-structure shown="Enabled" {
              disable-tunnel: ICP2-DO_Channel_Names."SW_LED - Ink Valve - R3" ("DO Channel") -> [w2190 w2204]
              disable-tunnel: w2181 -> [w2189 _]
              disable-tunnel: [w2188 w2192] -> w2180
              disable-tunnel: w2179 -> [w2187 w2206]
              disable-tunnel: "SW_LED - Ink Valve - R3" -> [w2186 w2191]
              disable-tunnel: w2177 -> [_ w2205]
              frame Disabled {
                n751 = call-dynamic "Set ICP2-DO Changed bit.vi"("error in (no error)"=w2187, "Value"=w2186, "DO Channel"=w2190, "IO in"=w2189) -> ("error out"=w2188:errorcluster)  [unwired: 6 in, 1 out]
              }
              frame Enabled {
                n752 = Format Into String(format string="%s", w2204) -> (resulting string=w2208:string)  [unwired: 2 in, 1 out]
                n753 = call "Set DO State (manual mode).vi"("error in (no error)"=w2206, "State"=w2191, "DO IOName"=w2208, "DAQ"=w2205) -> ("error out"=w2198:errorcluster, "DAQ"=w2199:refnum<class "DAQ.lvclass">)  [unwired: 6 in]
                n754 = Format Into String(format string="%s", error in=w2198, ICP2-DO_Channel_Names."Ink Flow Valve Open - R3" ("DO Channel")) -> (resulting string=w2203:string, error out=w2200:errorcluster)  [unwired: 1 in]
                n755 = call "Set DO State (automation mode).vi"("error in (no error)"=w2200, "State"=w2191, "DO IOName"=w2203, "DAQ"=w2199) -> ("error out"=w2193:errorcluster, "DAQ"=w2194:refnum<class "DAQ.lvclass">)  [unwired: 6 in]
                n756 = Format Into String(format string="%s", ICP2-DO_Channel_Names."Recirc Pump On - R3" ("DO Channel")) -> (resulting string=w2195:string)  [unwired: 2 in, 1 out]
                n757 = call "Set DO State (automation mode).vi"("error in (no error)"=w2193, "State"=w2191, "DO IOName"=w2195, "DAQ"=w2194) -> ("error out"=w2192:errorcluster)  [unwired: 6 in, 1 out]
              }
            }
          }
          event "SW_LED - Ink Valve - R4": Value Change {
            n758 = event-data() -> ()  [unwired: 1 in, 6 out]
            n759 = Unbundle By Name(w2214) -> ("DAQ"=w2209:refnum<class "DAQ.lvclass">, "IO"=w2213:refnum<class "IO.lvclass">)
            n760 = disable-structure shown="Enabled" {
              disable-tunnel: ICP2-DO_Channel_Names."SW_LED - Ink Valve - R4" ("DO Channel") -> [w2222 w2237]
              disable-tunnel: w2213 -> [w2221 _]
              disable-tunnel: [w2220 w2223] -> w2212
              disable-tunnel: w2211 -> [w2219 w2239]
              disable-tunnel: "SW_LED - Ink Valve - R4" -> [w2218 w2225]
              disable-tunnel: w2209 -> [_ w2238]
              frame Disabled {
                n761 = call-dynamic "Set ICP2-DO Changed bit.vi"("error in (no error)"=w2219, "Value"=w2218, "DO Channel"=w2222, "IO in"=w2221) -> ("error out"=w2220:errorcluster)  [unwired: 6 in, 1 out]
              }
              frame Enabled {
                n762 = Format Into String(format string="%s", w2237) -> (resulting string=w2241:string)  [unwired: 2 in, 1 out]
                n763 = call "Set DO State (manual mode).vi"("error in (no error)"=w2239, "State"=w2225, "DO IOName"=w2241, "DAQ"=w2238) -> ("error out"=w2231:errorcluster, "DAQ"=w2232:refnum<class "DAQ.lvclass">)  [unwired: 6 in]
                n764 = Format Into String(format string="%s", error in=w2231, ICP2-DO_Channel_Names."Ink Flow Valve Open - R4" ("DO Channel")) -> (resulting string=w2236:string, error out=w2233:errorcluster)  [unwired: 1 in]
                n765 = call "Set DO State (automation mode).vi"("error in (no error)"=w2233, "State"=w2225, "DO IOName"=w2236, "DAQ"=w2232) -> ("error out"=w2224:errorcluster, "DAQ"=w2227:refnum<class "DAQ.lvclass">)  [unwired: 6 in]
                n766 = Format Into String(format string="%s", error in=w2224, ICP2-DO_Channel_Names."Recirc Pump On - R4" ("DO Channel")) -> (resulting string=w2228:string, error out=w2226:errorcluster)  [unwired: 1 in]
                n767 = call "Set DO State (automation mode).vi"("error in (no error)"=w2226, "State"=w2225, "DO IOName"=w2228, "DAQ"=w2227) -> ("error out"=w2223:errorcluster)  [unwired: 6 in, 1 out]
              }
            }
          }
          event "SW_LED - Ink Valve - R5": Value Change {
            n768 = event-data() -> ()  [unwired: 1 in, 6 out]
            n769 = Unbundle By Name(w2247) -> ("DAQ"=w2242:refnum<class "DAQ.lvclass">, "IO"=w2246:refnum<class "IO.lvclass">)
            n770 = disable-structure shown="Enabled" {
              disable-tunnel: ICP2-DO_Channel_Names."SW_LED - Ink Valve - R5" ("DO Channel") -> [w2255 w2270]
              disable-tunnel: w2246 -> [w2254 _]
              disable-tunnel: [w2253 w2259] -> w2245
              disable-tunnel: w2244 -> [w2252 w2272]
              disable-tunnel: "SW_LED - Ink Valve - R5" -> [w2251 w2258]
              disable-tunnel: w2242 -> [_ w2271]
              frame Disabled {
                n771 = call-dynamic "Set ICP2-DO Changed bit.vi"("error in (no error)"=w2252, "Value"=w2251, "DO Channel"=w2255, "IO in"=w2254) -> ("error out"=w2253:errorcluster)  [unwired: 6 in, 1 out]
              }
              frame Enabled {
                n772 = Format Into String(format string="%s", w2270) -> (resulting string=w2274:string)  [unwired: 2 in, 1 out]
                n773 = call "Set DO State (manual mode).vi"("error in (no error)"=w2272, "State"=w2258, "DO IOName"=w2274, "DAQ"=w2271) -> ("error out"=w2264:errorcluster, "DAQ"=w2265:refnum<class "DAQ.lvclass">)  [unwired: 6 in]
                n774 = Format Into String(format string="%s", error in=w2264, ICP2-DO_Channel_Names."Ink Flow Valve Open - R5" ("DO Channel")) -> (resulting string=w2269:string, error out=w2266:errorcluster)  [unwired: 1 in]
                n775 = call "Set DO State (automation mode).vi"("error in (no error)"=w2266, "State"=w2258, "DO IOName"=w2269, "DAQ"=w2265) -> ("error out"=w2257:errorcluster, "DAQ"=w2260:refnum<class "DAQ.lvclass">)  [unwired: 6 in]
                n776 = Format Into String(format string="%s", error in=w2257, ICP2-DO_Channel_Names."Recirc Pump On - R5" ("DO Channel")) -> (resulting string=w2261:string, error out=w2256:errorcluster)  [unwired: 1 in]
                n777 = call "Set DO State (automation mode).vi"("error in (no error)"=w2256, "State"=w2258, "DO IOName"=w2261, "DAQ"=w2260) -> ("error out"=w2259:errorcluster)  [unwired: 6 in, 1 out]
              }
            }
          }
          event "SW_LED - Ink Valve - R6": Value Change {
            n778 = event-data() -> ()  [unwired: 1 in, 6 out]
            n779 = Unbundle By Name(w2280) -> ("DAQ"=w2275:refnum<class "DAQ.lvclass">, "IO"=w2279:refnum<class "IO.lvclass">)
            n780 = disable-structure shown="Enabled" {
              disable-tunnel: ICP2-DO_Channel_Names."SW_LED - Ink Valve - R6" ("DO Channel") -> [w2288 w2302]
              disable-tunnel: w2279 -> [w2287 _]
              disable-tunnel: [w2286 w2290] -> w2278
              disable-tunnel: w2277 -> [w2285 w2304]
              disable-tunnel: "SW_LED - Ink Valve - R6" -> [w2284 w2289]
              disable-tunnel: w2275 -> [_ w2303]
              frame Disabled {
                n781 = call-dynamic "Set ICP2-DO Changed bit.vi"("error in (no error)"=w2285, "Value"=w2284, "DO Channel"=w2288, "IO in"=w2287) -> ("error out"=w2286:errorcluster)  [unwired: 6 in, 1 out]
              }
              frame Enabled {
                n782 = Format Into String(format string="%s", w2302) -> (resulting string=w2306:string)  [unwired: 2 in, 1 out]
                n783 = call "Set DO State (manual mode).vi"("error in (no error)"=w2304, "State"=w2289, "DO IOName"=w2306, "DAQ"=w2303) -> ("error out"=w2297:errorcluster, "DAQ"=w2296:refnum<class "DAQ.lvclass">)  [unwired: 6 in]
                n784 = Format Into String(format string="%s", error in=w2297, ICP2-DO_Channel_Names."Ink Flow Valve Open - R6" ("DO Channel")) -> (resulting string=w2301:string, error out=w2300:errorcluster)  [unwired: 1 in]
                n785 = call "Set DO State (automation mode).vi"("error in (no error)"=w2300, "State"=w2289, "DO IOName"=w2301, "DAQ"=w2296) -> ("error out"=w2291:errorcluster, "DAQ"=w2292:refnum<class "DAQ.lvclass">)  [unwired: 6 in]
                n786 = Format Into String(format string="%s", ICP2-DO_Channel_Names."Recirc Pump On - R6" ("DO Channel")) -> (resulting string=w2293:string)  [unwired: 2 in, 1 out]
                n787 = call "Set DO State (automation mode).vi"("error in (no error)"=w2291, "State"=w2289, "DO IOName"=w2293, "DAQ"=w2292) -> ("error out"=w2290:errorcluster)  [unwired: 6 in, 1 out]
              }
            }
          }
          event "Recirc Pump On - R1": Value Change {
            n788 = event-data() -> ()  [unwired: 1 in, 6 out]
            n789 = Unbundle By Name(w2312) -> ("DAQ"=w2307:refnum<class "DAQ.lvclass">, "IO"=w2311:refnum<class "IO.lvclass">)
            n790 = disable-structure shown="Enabled" {
              disable-tunnel: ICP2-DO_Channel_Names."Recirc Pump On - R1" ("DO Channel") -> [w2320 w2336]
              disable-tunnel: w2311 -> [w2319 _]
              disable-tunnel: [w2318 w2321] -> w2310
              disable-tunnel: w2309 -> [w2317 w2337]
              disable-tunnel: "Recirc Pump On - R1" -> [w2316 w2324]
              disable-tunnel: w2307 -> [_ w2335]
              frame Disabled {
                n791 = call-dynamic "Set ICP2-DO Changed bit.vi"("error in (no error)"=w2317, "Value"=w2316, "DO Channel"=w2320, "IO in"=w2319) -> ("error out"=w2318:errorcluster)  [unwired: 6 in, 1 out]
              }
              frame Enabled {
                n792 = Format Into String(format string="%s", w2336) -> (resulting string=w2339:string)  [unwired: 2 in, 1 out]
                n793 = call "Set DO State (manual mode).vi"("error in (no error)"=w2337, "State"=w2324, "DO IOName"=w2339, "DAQ"=w2335) -> ("error out"=w2322:errorcluster, "DAQ"=w2331:refnum<class "DAQ.lvclass">)  [unwired: 6 in]
                n794 = Format Into String(format string="%s", error in=w2322, ICP2-DO_Channel_Names."SW_LED - Ink Valve - R1" ("DO Channel")) -> (resulting string=w2334:string, error out=w2330:errorcluster)  [unwired: 1 in]
                n795 = call "Set DO State (automation mode).vi"("error in (no error)"=w2330, "State"=w2324, "DO IOName"=w2334, "DAQ"=w2331) -> ("error out"=w2323:errorcluster, "DAQ"=w2326:refnum<class "DAQ.lvclass">)  [unwired: 6 in]
                n796 = Format Into String(format string="%s", error in=w2323, ICP2-DO_Channel_Names."Ink Flow Valve Open - R1" ("DO Channel")) -> (resulting string=w2327:string, error out=w2329:errorcluster)  [unwired: 1 in]
                n797 = call "Set DO State (automation mode).vi"("error in (no error)"=w2329, "State"=w2324, "DO IOName"=w2327, "DAQ"=w2326) -> ("error out"=w2321:errorcluster)  [unwired: 6 in, 1 out]
              }
            }
          }
          event "Recirc Pump On - R2": Value Change {
            n798 = event-data() -> ()  [unwired: 1 in, 6 out]
            n799 = Unbundle By Name(w2345) -> ("DAQ"=w2340:refnum<class "DAQ.lvclass">, "IO"=w2344:refnum<class "IO.lvclass">)
            n800 = disable-structure shown="Enabled" {
